vi "CRYMsgs Curves Gen Construct.vi"(4 "Interface type":u16, 5 "GPIB func":u16, 6 "Step name":string, 7 "Type":u16, 8 "RS232 func":u16, 9 "Operation":i32, 10 "Numeric?":bool, 11 "Dialog?":bool) -> (3 "Curves generated":string[](array[string]))   [LabVIEW 2013]
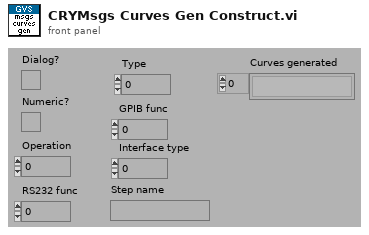
[diagram p1: front panel]
types:
  T1 = typedef "CRYData Cluster.ctl" = cluster{"Name":string, "Curve":cluster{"x":dbl, "y":dbl, "z":dbl}[], "X data":u16, "Y data":u16, "Z data":u16, "X axis":u16, "Y axis":u16, "Z axis":u16, "X unit":string, "Y unit":string, "Z unit":string, "X dB ref":dbl, "Y dB ref":dbl, "Z dB ref":dbl, "single val":bool, "protected":bool, "display X":bool, "display Y":bool, "display Z":bool, "Test Info":string, "Step No.":i32, "Plot Settings":cluster{"Color":u32, "Interpolation":u8, "Point Style":u8, "Line Style":u8, "Point Color":u32, "Line Width":u8, "Bar Plot Style":u8, "Fill To":i16}, "AutoProtect":bool}
  T2 = typedef "CRYResult Cluster.ctl" = cluster{"Name":string, "Margin":dbl, "unit":string, "Verdict":bool, "Limit":string, "Max/Min":string, "protected":bool, "Step No.":i32, "Test Info":string, "AutoProtect":bool}
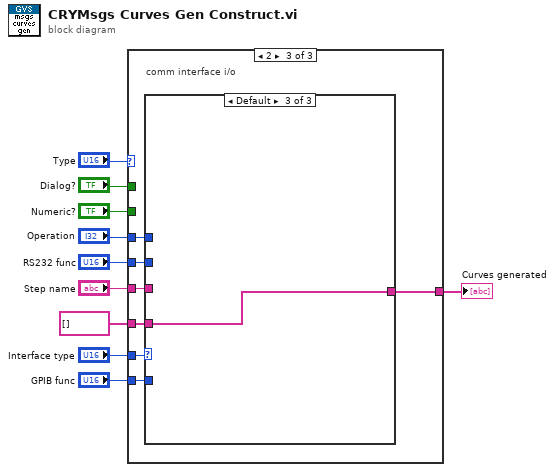
[diagram p0: block diagram]
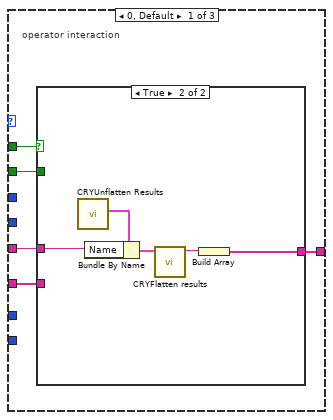
[diagram p2: hidden frame]
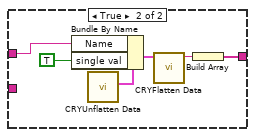
[diagram p4: hidden frame]
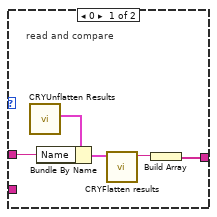
[diagram p6: hidden frame]
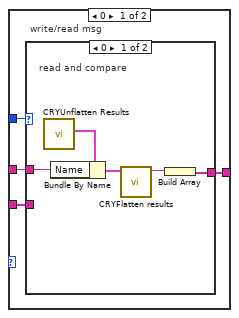
[diagram p8: hidden frame]
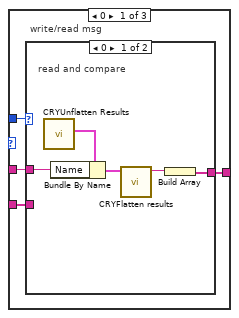
[diagram p11: hidden frame]
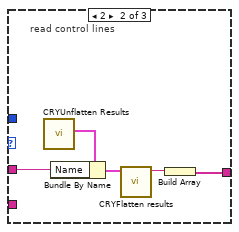
[diagram p13: hidden frame]
diagram:
  n1 = case shown="2" "Type" {
    tunnel: "Dialog?" -> [w15 _ _]
    tunnel: "Numeric?" -> [w12 _ _]
    tunnel: "Step name" -> [w14 w33 w45]
    tunnel: [w13 w34 w44] -> w4
    tunnel: "Operation" -> [_ w35 w46]
    tunnel: string[] [] ("Curves generated") -> [w11 w32 w43]
    tunnel: "Interface type" -> [_ _ w48]
    tunnel: "GPIB func" -> [_ _ w47]
    tunnel: "RS232 func" -> [_ _ w42]
    frame 0, Default {
      # "operator interaction"
      n2 = case shown="True" w15 {
        tunnel: w14 -> [w18 w30]
        tunnel: [w17 w28] -> w13
        tunnel: w12 -> [w19 _]
        tunnel: w11 -> [w16 _]
        frame False {
          n3 = case shown="False" w19 {
            tunnel: w18 -> [_ w22]
            tunnel: [w20 w21] -> w17
            tunnel: w16 -> [w20 _]
            frame False {
            }
            frame True {
              n4 = call "CRYUnflatten Data.vi"() -> ("Datum"=w25:T1)  [unwired: 9 in, 2 out]
              n5 = Bundle By Name(cluster=w25, "Name"=w22, "single val"=TRUE ("Bundle Element")) -> (w26:T1)
              n6 = call "CRYFlatten Data.vi"("Datum"=w26) -> ("Data flattened"=w23:string)  [unwired: 10 in]
              n7 = Build Array(w23) -> (w21:string[])
            }
          }
        }
        frame True {
          n8 = call "CRYUnflatten Results.vi"() -> ("Result"=w31:T2)  [unwired: 9 in, 2 out]
          n9 = Bundle By Name(cluster=w31, "Name"=w30) -> (w27:T2)
          n10 = call "CRYFlatten results.vi"("Result in"=w27) -> ("Flatten Result"=w29:string)  [unwired: 10 in]
          n11 = Build Array(w29) -> (w28:string[])
        }
      }
    }
    frame 1 {
      # "digital i/o"
      n12 = case shown="Default" w35 {
        tunnel: [w37 w41] -> w34
        tunnel: w33 -> [w38 _]
        tunnel: w32 -> [_ w41]
        frame 0 {
          # "read and compare"
          n13 = call "CRYUnflatten Results.vi"() -> ("Result"=w40:T2)  [unwired: 9 in, 2 out]
          n14 = Bundle By Name(cluster=w40, "Name"=w38) -> (w36:T2)
          n15 = call "CRYFlatten results.vi"("Result in"=w36) -> ("Flatten Result"=w39:string)  [unwired: 10 in]
          n16 = Build Array(w39) -> (w37:string[])
        }
        frame Default {
        }
      }
    }
    frame 2 {
      # "comm interface i/o"
      n17 = case shown="Default" w48 {
        tunnel: w47 -> [w53 _ _]
        tunnel: w46 -> [w52 w69 _]
        tunnel: w45 -> [w51 w68 _]
        tunnel: [w50 w67 w86] -> w44
        tunnel: w43 -> [w49 w66 w86]
        tunnel: w42 -> [_ w65 _]
        frame 0 {
          # "GPIB"
          n18 = case shown="Default" w53 {
            tunnel: w52 -> [w57 _]
            tunnel: w51 -> [w56 _]
            tunnel: [w55 w64] -> w50
            tunnel: w49 -> [w54 w64]
            frame 0 {
              # "write/read msg"
              n19 = case shown="0" w57 {
                tunnel: w56 -> [w60 _]
                tunnel: [w59 w63] -> w55
                tunnel: w54 -> [_ w63]
                frame 0 {
                  # "read and compare"
                  n20 = call "CRYUnflatten Results.vi"() -> ("Result"=w61:T2)  [unwired: 9 in, 2 out]
                  n21 = Bundle By Name(cluster=w61, "Name"=w60) -> (w58:T2)
                  n22 = call "CRYFlatten results.vi"("Result in"=w58) -> ("Flatten Result"=w62:string)  [unwired: 10 in]
                  n23 = Build Array(w62) -> (w59:string[])
                }
                frame Default {
                }
              }
            }
            frame Default {
            }
          }
        }
        frame 1 {
          # "RS-232"
          n24 = case shown="Default" w65 {
            tunnel: w69 -> [w73 _ _]
            tunnel: w68 -> [w72 w84 _]
            tunnel: [w71 w83 w85] -> w67
            tunnel: w66 -> [w70 _ w85]
            frame 0 {
              # "write/read msg"
              n25 = case shown="0" w73 {
                tunnel: w72 -> [w76 _]
                tunnel: [w75 w79] -> w71
                tunnel: w70 -> [_ w79]
                frame 0 {
                  # "read and compare"
                  n26 = call "CRYUnflatten Results.vi"() -> ("Result"=w77:T2)  [unwired: 9 in, 2 out]
                  n27 = Bundle By Name(cluster=w77, "Name"=w76) -> (w74:T2)
                  n28 = call "CRYFlatten results.vi"("Result in"=w74) -> ("Flatten Result"=w78:string)  [unwired: 10 in]
                  n29 = Build Array(w78) -> (w75:string[])
                }
                frame Default {
                }
              }
            }
            frame 2 {
              # "read control lines"
              n30 = call "CRYUnflatten Results.vi"() -> ("Result"=w81:T2)  [unwired: 9 in, 2 out]
              n31 = Bundle By Name(cluster=w81, "Name"=w84) -> (w80:T2)
              n32 = call "CRYFlatten results.vi"("Result in"=w80) -> ("Flatten Result"=w82:string)  [unwired: 10 in]
              n33 = Build Array(w82) -> (w83:string[])
            }
            frame Default {
            }
          }
        }
        frame Default {
        }
      }
    }
  }
  "Curves generated" <- w4
